vi "Link_Create Linker files.vi"(7 "Run Data":T1={"Target Folder"=path "", "Menu Folder"=path "", "Active Folder"=path "", "Config"={"Main"={"Menu Folder"="", "Re-Create Menu Folder?"=FALSE, "Allow mnu replace?"=FALSE, "Relative Link Target"="", "Auto Link?"=FALSE}, "File Filter"={"Exclude Prefixes"=[], "Ignore Names"=[], "Include Extensions"=[], "Exclude Postfixes"=[]}, "Folder Filter"={"Exclude Prefixes"=[], "Ignore Names"=[]}, "File Name Edit"={"Pre Split String"="", "Post Split String"="", "Deletion Strings"=[]}, "Folder Name Edit"={"Pre Split String"="", "Post Split String"="", "Deletion Strings"=[]}, "Folder Icon Map"={}, "Default Palette Data"={"Display Name Override"="", "View Format"=2, "Palette Width"=0, "Help Tag"="", "Help File Path"=path "", "Palette Description"=""}, "Default File Data"={"Display Name Override"="", "Place VI Contents?"=FALSE}, "Palette Override map"={}, "File Override map"={}}} {"Config"."Default Palette Data"."View Format" items=["Icons", "Text", "Icons and Text"]}, 8 "error in (no error)":errorcluster, 10 "Link Target Root Override (\"\")":path, 11 "Created mnu file paths":path[](array[path])) -> (0 "error out":errorcluster, 1 "Link files created?":bool, 2 "Unlinker":path, 3 "Linker":path)   [LabVIEW 2019, in "AutoMenuCreator.lvlib"]
uses:
  AutoMenuCreator.lvlib
  Ctl/Ctl_Run Data.ctl
  Ctl/Ctl_Config.ctl
  Ctl/Ctl_Config_Main.ctl
  Ctl/Ctl_Config_File Filter.ctl
  Ctl/Ctl_Config_Folder Filter.ctl
  Ctl/Ctl_Config_Name Edit.ctl
  Ctl/Ctl_Config_Folder Icon Map.ctl
  Ctl/Ctl_Config_Palette Data.ctl
  <vilib>/Palette API/Palette Menu/Public Type Define/View Format.ctl
  Ctl/Ctl_Config_File Data.ctl
  <vilib>/Palette API/Palette Menu/Palette Menu.lvlib
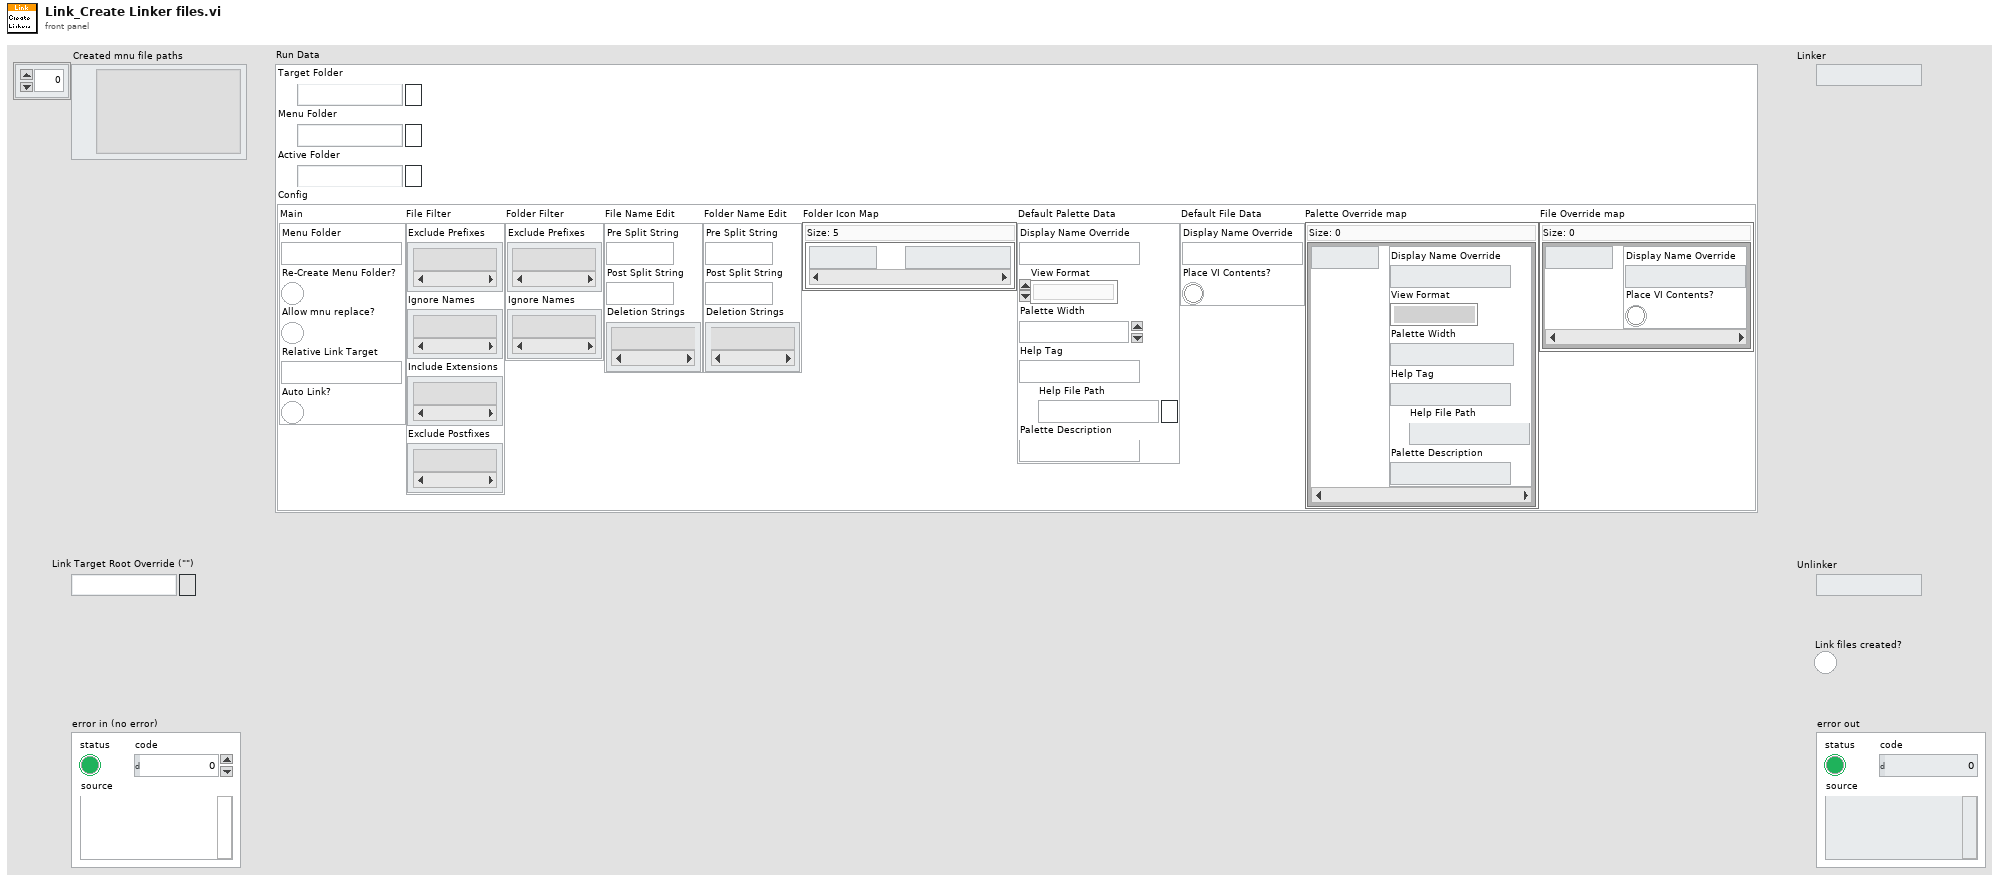
[diagram p1: front panel]
types:
  T1 = typedef "AutoMenuCreator.lvlib/Ctl_Run Data.ctl" = cluster{"Target Folder":path, "Menu Folder":path, "Active Folder":path, "Config":T2}
  T2 = typedef "AutoMenuCreator.lvlib/Ctl_Config.ctl" = cluster{"Main":T3, "File Filter":T4, "Folder Filter":T5, "File Name Edit":T6, "Folder Name Edit":T6, "Folder Icon Map":T7, "Default Palette Data":T8, "Default File Data":T10, "Palette Override map":map{string, T8}, "File Override map":map{string, T10}}
  T3 = typedef "AutoMenuCreator.lvlib/Ctl_Config_Main.ctl" = cluster{"Menu Folder":string, "Re-Create Menu Folder?":bool, "Allow mnu replace?":bool, "Relative Link Target":string, "Auto Link?":bool}
  T4 = typedef "AutoMenuCreator.lvlib/Ctl_Config_File Filter.ctl" = cluster{"Exclude Prefixes":string[], "Ignore Names":string[], "Include Extensions":string[], "Exclude Postfixes":string[]}
  T5 = typedef "AutoMenuCreator.lvlib/Ctl_Config_Folder Filter.ctl" = cluster{"Exclude Prefixes":string[], "Ignore Names":string[]}
  T6 = typedef "AutoMenuCreator.lvlib/Ctl_Config_Name Edit.ctl" = cluster{"Pre Split String":string, "Post Split String":string, "Deletion Strings":string[]}
  T7 = typedef "AutoMenuCreator.lvlib/Ctl_Config_Folder Icon Map.ctl" = map{string, path}
  T8 = typedef "AutoMenuCreator.lvlib/Ctl_Config_Palette Data.ctl" = cluster{"Display Name Override":string, "View Format":T9, "Palette Width":i16, "Help Tag":string, "Help File Path":path, "Palette Description":string}
  T9 = typedef "Palette Menu.lvlib/View Format.ctl" = u16
  T10 = typedef "AutoMenuCreator.lvlib/Ctl_Config_File Data.ctl" = cluster{"Display Name Override":string, "Place VI Contents?":bool}
  T11 = enum16{"open", "replace", "create", "open or create", "replace or create", "replace or create with confirmation"}
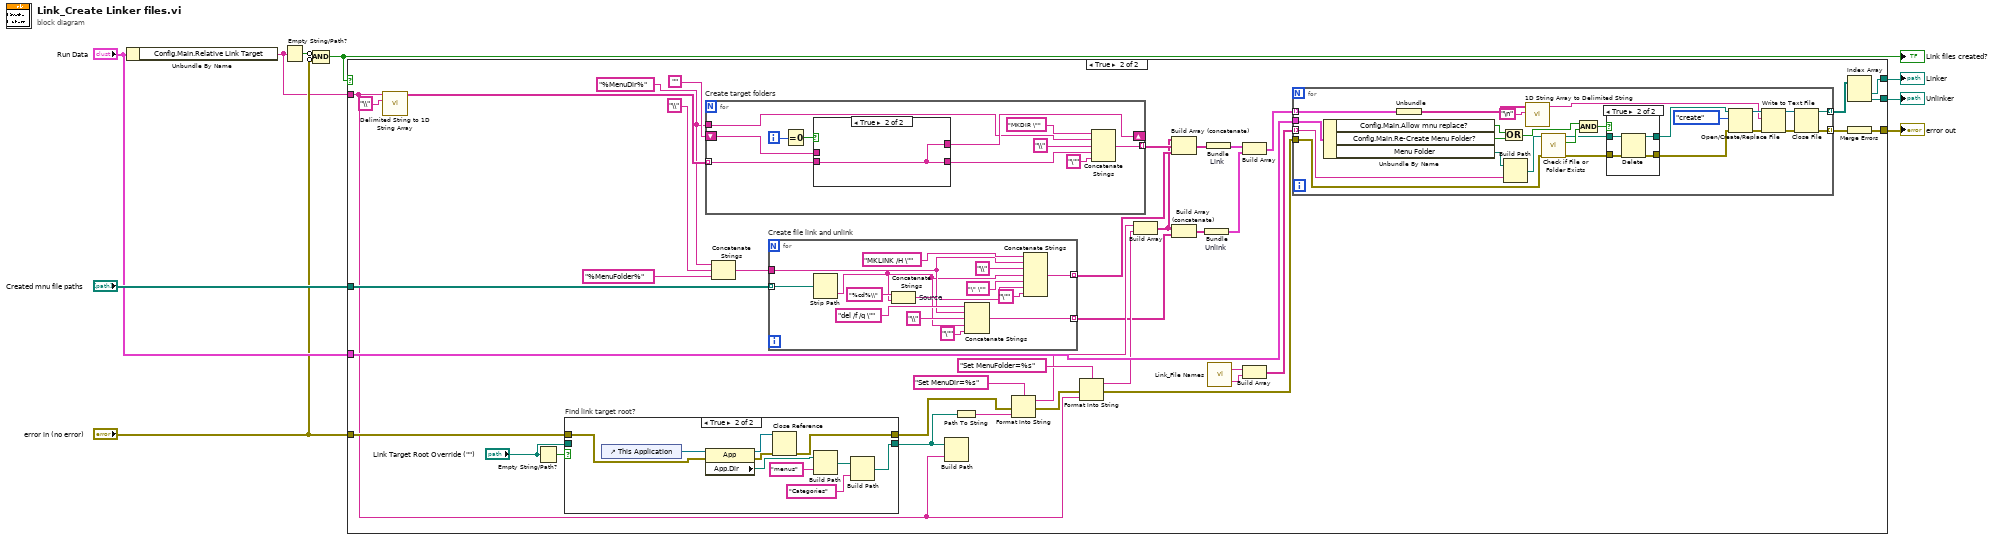
[diagram p0: block diagram]
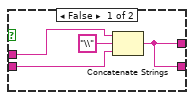
[diagram p4: hidden frame]
diagram:
  n1 = Unbundle By Name("Run Data") -> ("Config.Main.Relative Link Target"=w4:string)
  n2 = Empty String/Path?(string/path=w4) -> (empty?=w7:bool)
  n3 = Compound Arithmetic op=AND(invert w7, invert "error in (no error)") -> (w5:bool)
  "Link files created?" <- w5
  n4 = case shown="True" w5 {
    tunnel: "Created mnu file paths" -> [_ w49]
    tunnel: "Run Data" -> [_ w33]
    tunnel: "error in (no error)" -> [w10 w46]
    tunnel: w4 -> [_ w23]
    tunnel: [w10 w31] -> w3
    tunnel: [_ w29] -> w2
    tunnel: [_ w28] -> w1
    frame False {
    }
    frame True {
      w13 = "%MenuDir%"
      n5 = call <vilib>:"Delimited String to 1D String Array.vi"("delimiter"="\\", "delimited string"=w23) -> ("string array"=w44:string[])  [unwired: 9 in]
      n6 = Empty String/Path?(string/path="Link Target Root Override (\"\")") -> (empty?=w48:bool)
      n7 = case "Find link target root?" shown="True" w48 {
        tunnel: [w98 w101] -> w27
        tunnel: "Link Target Root Override (\"\")" -> [w98 _]
        tunnel: w46 -> [w97 w100]
        tunnel: [w97 w99] -> w21
        frame False {
        }
        frame True {
          n8 = control-ref of="This Application"() -> (w108:refnum<vi>)
          n9 = property class="App"(reference=w108, error in=w100) -> (reference out=w106:refnum<vi>, error out=w107:errorcluster, "App.Dir"=w105:path)
          n10 = Close Reference(reference=w106, error in (no error)=w107) -> (error out=w99:errorcluster)
          n11 = Build Path(base path=w105, name or relative path="menus") -> (appended path=w103:path)
          n12 = Build Path(base path=w103, name or relative path="Categories") -> (appended path=w101:path)
        }
      }
      n13 = for "Create target folders" {
        tunnel: w44 -> [w89] mode=indexing
        shift-right: [w87] -> _
        shift-left: "" -> [w88]
        tunnel: [w81] -> w42 mode=indexing
        tunnel: w13 -> [w85]
        i -> [w91]
        n14 = Equal To 0?(x=w91) -> (x = 0?=w90:bool)
        n15 = case shown="True" w90 {
          tunnel: [w92 w96] -> w83
          tunnel: w89 -> [w93 w96]
          tunnel: w88 -> [w95 _]
          tunnel: [w92 w96] -> w87
          frame False {
            n16 = Concatenate Strings(w95, "\\" ("string"), w93) -> (w92:string)
          }
          frame True {
          }
        }
        n17 = Concatenate Strings("MKDIR \"" ("string"), w85, "\\" ("string"), w83, "\"" ("string")) -> (w81:string)
      }
      n18 = Concatenate Strings(w13, "\\" ("string"), "%MenuFolder%") -> (w19:string)
      n19 = for "Create file link and unlink" {
        tunnel: w49 -> [w122] mode=indexing
        tunnel: [w110] -> w41 mode=indexing
        tunnel: [w117] -> w15 mode=indexing
        tunnel: w19 -> [w115]
        n20 = Strip Path(path=w122) -> (name=w109:string)  [unwired: 1 out]
        n21 = Concatenate Strings "Source"("%cd%\\", w109) -> (w112:string)
        n22 = Concatenate Strings("del /f /q \"" ("string"), w115, "\\" ("string"), w109, "\"" ("string")) -> (w117:string)
        n23 = Concatenate Strings("MKLINK /H \"" ("string"), w115, "\\" ("string"), w109, "\" \"" ("string"), w112, "\"" ("string")) -> (w110:string)
      }
      n24 = Build Path(base path=w27, name or relative path=w23) -> ()  [unwired: 1 out]
      n25 = Path To String(path=w27) -> (string=w25:string)
      n26 = Format Into String(format string="Set MenuDir=%s", error in=w21, w25) -> (resulting string=w18:string, error out=w22:errorcluster)  [unwired: 1 in]
      n27 = Format Into String(format string="Set MenuFolder=%s", error in=w22, w23) -> (resulting string=w17:string, error out=w11:errorcluster)  [unwired: 1 in]
      n28 = Build Array(w18, w17) -> (w16:string[])
      n29 = Build Array (concatenate)(w16, w42, w41) -> (w40:string[])
      n30 = Build Array (concatenate)(w16, w15) -> (w14:string[])
      n31 = Bundle "Unlink"(w14) -> (w38:cluster{string[]})  [unwired: 1 in]
      n32 = Bundle "Link"(w40) -> (w39:cluster{string[]})  [unwired: 1 in]
      n33 = call "Link_File Names.vi"() -> ("Unlink file name"=w35:string, "Link file name"=w36:string)  [unwired: 2 in]
      n34 = Build Array(w39, w38) -> (w37:cluster{string[]}[])
      n35 = Build Array(w36, w35) -> (w34:string[])
      n36 = for {
        tunnel: w11 -> [w50]
        tunnel: w37 -> [w74] mode=indexing
        tunnel: w34 -> [w69] mode=indexing
        tunnel: w33 -> [w72]
        tunnel: [w53] -> w32 mode=indexing
        tunnel: [w52] -> w30 mode=indexing
        n37 = Unbundle By Name(w72) -> ("Config.Main.Allow mnu replace?"=w71:bool, "Config.Main.Re-Create Menu Folder?"=w73:bool, "Menu Folder"=w70:path)
        n38 = Unbundle(w74) -> (w60:string[])
        n39 = Or(x=w71, y=w73) -> (x .or. y?=w66:bool)
        n40 = Build Path(base path=w70, name or relative path=w69) -> (appended path=w68:path)
        n41 = call <vilib>:"1D String Array to Delimited String.vi"("delimiter"="\n", "string array"=w60) -> ("delimited string"=w57:string)  [unwired: 9 in]
        n42 = call <vilib>:"Check if File or Folder Exists.vi"("error in (no error)"=w50, "path"=w68) -> ("error out"=w51:errorcluster, "file or folder exists?"=w67:bool, "dup path"=w64:path)  [unwired: 7 in]
        n43 = And(x=w66, y=w67) -> (x .and. y?=w65:bool)
        n44 = case shown="True" w65 {
          tunnel: [w76 w79] -> w61
          tunnel: w51 -> [w76 w80]
          tunnel: w64 -> [w75 w78]
          tunnel: [w75 w77] -> w63
          frame False {
          }
          frame True {
            n45 = Delete(path (use dialog)=w78, error in=w80) -> (deleted path=w77:path, error out=w79:errorcluster)  [unwired: 3 in, 1 out]
          }
        }
        n46 = Open/Create/Replace File(file path (use dialog)=w63, error in=w61, operation (0:open)=T11."create") -> (refnum out=w58:refnum<file>, error out=w56:errorcluster)  [unwired: 3 in, 1 out]
        n47 = Write to Text File(file (use dialog)=w58, text=w57, error in=w56) -> (refnum out=w55:refnum<file>, error out=w54:errorcluster)  [unwired: 1 in, 1 out]
        n48 = Close File(refnum=w55, error in=w54) -> (path=w52:path, error out=w53:errorcluster)
      }
      n49 = Index Array(array=w30) -> (element #1=w29:path, element #2=w28:path)  [unwired: 2 in]
      n50 = Merge Errors(w32) -> (w31:errorcluster)
    }
  }
  "error out" <- w3
  "Linker" <- w2
  "Unlinker" <- w1
